vi "Data handler-AOL Zstack.vi"(4 "Save image":bool, 6 "Single Frame Data":T2, 8 "error in (no error)":errorcluster, 9 "Live graph data queue in":T1, 10 "Logging queue element in":T5={"Imaging Protocol"=enum."Live Imaging", "Number of Trials"=0, "Frame Size"=512, "# Averaged frames"=0, "Dwell time (us)"=0.0, "Index of Z-plane"=0, "Timelapse?"=FALSE, "Logging process is active"=FALSE, "Speed logging enabled"=FALSE, "tdms file ref"=refnum, "path"=path "", "Trial Number"=0, "Expected # points acquired"=FALSE, "Manually stopped"=FALSE, "Last trial"=FALSE, "Ch0 data"=[], "Ch1 data"=[], "Image Time"=[], "Continuous Time"=[], "Points acquired"={"Ch0 last trial"=0, "Ch1 last trial"=0, "All trials"=0}, "HW Timings File"=refnum} {"Frame Size" items=["100X100"=100, "128X128"=128, "200X200"=200, "256X256"=256, "512X512"=512, "1024x1024"=1024, "2048x2048"=2048]; "Dwell time (us)" format="%#.6g"}, 11 "Image array":T3) -> (0 "error out":errorcluster)   [LabVIEW 2017]
uses:
  Typedefs/Logging queue element.ctl
  Typedefs/Imaging Protocols enum.ctl
  Typedefs/Frame Size.ctl
  Typedefs/Acquired points count.ctl
  User Interface/Queue/Live graphs queue/Typedefs/Live imaging queue element.ctl
  <vilib>/vision/Image Controls.llb/IMAQ Image.ctl
  Typedefs/Frame data dual cluster.ctl
  User Interface/Typedefs/Live graph data queue ref.ctl
  Typedefs/Subpanel close request.ctl
  Typedefs/Top level VI states.ctl
  Global Variables/General Globals.vi
panel:
  out "Subpanel is closed / Proceed":bool
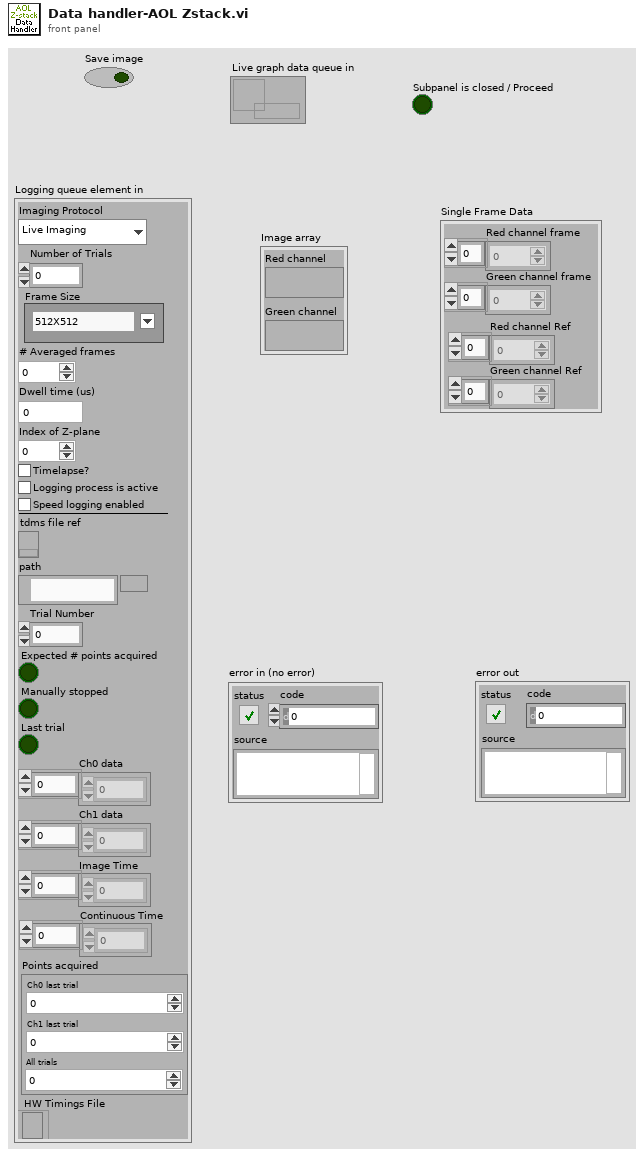
[diagram p1: front panel]
types:
  T1 = typedef "Live graph data queue ref.ctl" = refnum<queue>
  T2 = typedef "Frame data dual cluster.ctl" = cluster{"Red channel frame":dbl[], "Green channel frame":dbl[], "Red channel Ref":dbl[], "Green channel Ref":dbl[]}
  T3 = typedef "Live imaging queue element.ctl" = cluster{"Red channel":T4, "Green channel":T4}
  T4 = typedef "IMAQ Image.ctl" = refnum<image>
  T5 = typedef "Logging queue element.ctl" = cluster{"Imaging Protocol":T6, "Number of Trials":u16, "Frame Size":T7, "# Averaged frames":u16, "Dwell time (us)":dbl, "Index of Z-plane":i32, "Timelapse?":bool, "Logging process is active":bool, "Speed logging enabled":bool, "tdms file ref":refnum<k34>, "path":path, "Trial Number":i32, "Expected # points acquired":bool, "Manually stopped":bool, "Last trial":bool, "Ch0 data":u32[], "Ch1 data":u32[], "Image Time":u64[], "Continuous Time":u64[], "Points acquired":T8, "HW Timings File":refnum<file>}
  T6 = typedef "Imaging Protocols enum.ctl" = enum16{"AOL Z-Stack", "Motor Z Stack", "Functional Acquisition", "Single Plane Acquisition", "Volume Acquisition", "Live Imaging", "Live Plane Imaging", "Live Volume Imaging"}
  T7 = typedef "Frame Size.ctl" = u16
  T8 = typedef "Acquired points count.ctl" = cluster{"Ch0 last trial":u64, "Ch1 last trial":u64, "All trials":u64}
  T9 = typedef "Subpanel close request.ctl" = enum16{"Request subpanel close", "Just check subpanel is closed"}
  T10 = typedef "Top level VI states.ctl" = enum16{"None", "Initialise UI", "<STACK PROTOCOL STATES>", "AOL Zstack-START", "AOL Zstack-STOP", "Motor Zstack-START", "Motor Zstack-STOP", "<ACQUISITION PROTOCOL STATES> ", "Functional Acquisition-START", "Functional Acquisition-STOP", "Single Plane Acquisition-START", "Single Plane Acquisition-STOP", "Volume Acquisition-START", "Volume Acquisition-STOP", "<LIVE IMAGING PROTOCOL STATES>", "Live Imaging-START", "Live Imaging-STOP", "Live Plane Imaging-START", "Live Plane Imaging-STOP", "Live Volume Imaging-START", "Live Volume Imaging-STOP", "<MOVEMENT CORRECTION PROTOCOL STATES>", "EXIT"}
  T11 = enum16{"open", "replace", "create", "open or create", "replace or create", "replace or create with confirmation"}
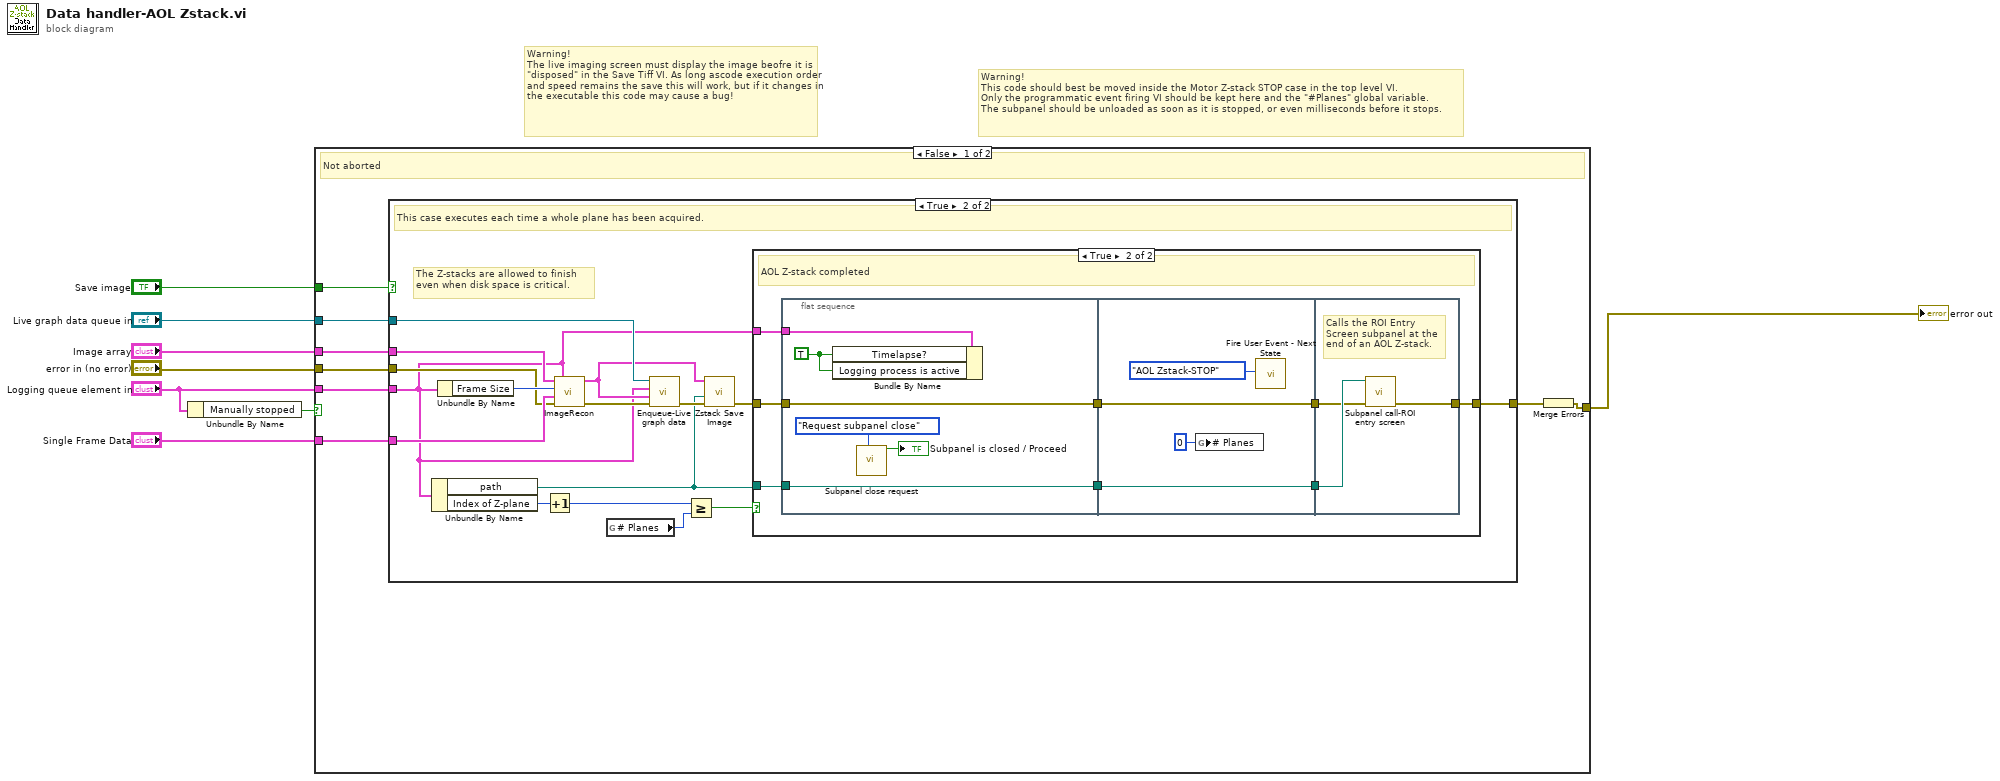
[diagram p0: block diagram]
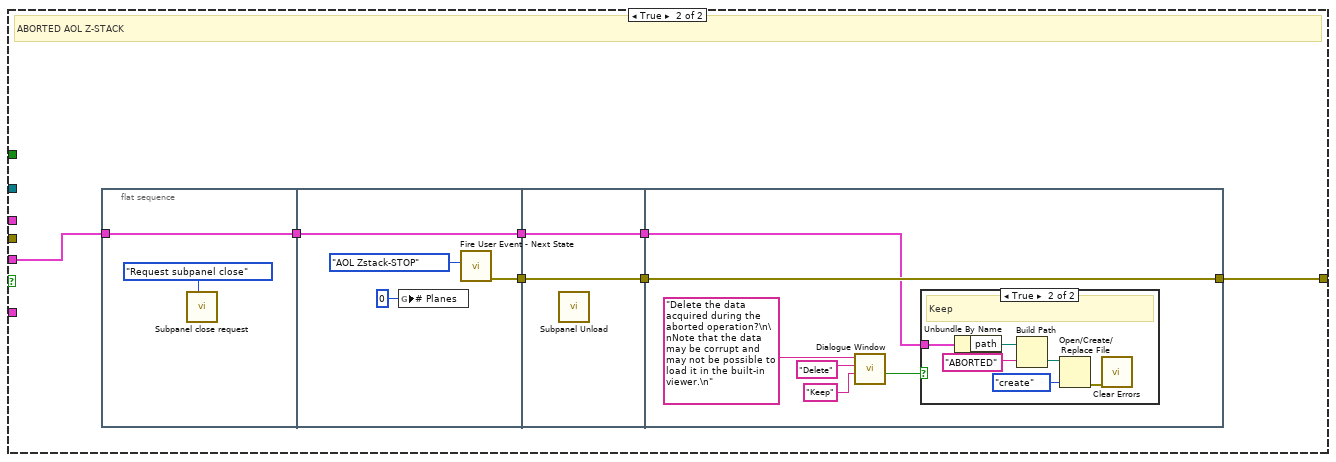
[diagram p4: hidden frame]
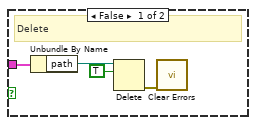
[diagram p5: hidden frame]
diagram:
  # "Warning!\nThe live imaging screen must display the image beofre it is \"disposed\" in the Save Tiff VI. As long ascode execution order and speed remains the save this will work, but if it changes in the executable this code may cause a bug!"
  # "Warning!\nThis code should best be moved inside the Motor Z-stack STOP case in the top level VI.\nOnly the programmatic event firing VI should be kept here and the \"#Planes\" global variable.\nThe subpanel should be unloaded as soon as it is stopped, or even milliseconds before it stops."
  n1 = Unbundle By Name("Logging queue element in") -> ("Manually stopped"=w1:bool)
  n2 = case shown="False" w1 {
    tunnel: "Save image" -> [w15 _]
    tunnel: "error in (no error)" -> [w14 _]
    tunnel: "Live graph data queue in" -> [w13 _]
    tunnel: "Image array" -> [w12 _]
    tunnel: "Single Frame Data" -> [w11 _]
    tunnel: [w10 w61] -> w3
    tunnel: "Logging queue element in" -> [w9 w58]
    frame False {
      # "Not aborted"
      n3 = case shown="True" w15 {
        tunnel: [_ w32] -> w16
        tunnel: w12 -> [_ w30]
        tunnel: w9 -> [_ w18]
        tunnel: w11 -> [_ w27]
        tunnel: w14 -> [_ w26]
        tunnel: w13 -> [_ w25]
        frame False {
          # "Acquisition of the current plane has not completed. Plane is incomplete."
        }
        frame True {
          # "The Z-stacks are allowed to finish even when disk space is critical."
          # "This case executes each time a whole plane has been acquired."
          n4 = Unbundle By Name(w18) -> ("path"=w22:path, "Index of Z-plane"=w28:i32)
          n5 = Unbundle By Name(w18) -> ("Frame Size"=w29:T7)
          n6 = Increment(x=w28) -> (x+1=w31:i32)
          n7 = call "ImageRecon.vi"("Logging queue element in"=w18, "Error In"=w26, "Data"=w27, "Frame Size"=w29, "Image Array (in)"=w30) -> ("Error Out"=w21:errorcluster, "Image Array(out)"=w20:T3)  [unwired: 3 in, 2 out]
          n8 = global read "General Globals.vi" "# Planes"() -> (w19:i32)
          n9 = call "Enqueue-Live graph data.vi"("error in (no error)"=w21, "Element to queue"=w20, "Logging queue element"=w18, "Live graph data queue in"=w25) -> ("error out"=w24:errorcluster)  [unwired: 6 in, 1 out]
          n10 = Greater Or Equal?(x=w31, y=w19) -> (x >= y?=w17:bool)
          n11 = call "Zstack Save Image.vi"("error in (no error)"=w24, "Dataset base-path"=w22, "Image Array"=w20) -> ("error out"=w23:errorcluster)  [unwired: 8 in]
          n12 = case shown="True" w17 {
            tunnel: w23 -> [w33 w39]
            tunnel: w22 -> [_ w41]
            tunnel: [w33 w40] -> w32
            tunnel: w18 -> [_ w34]
            frame False {
            }
            frame True {
              # "AOL Z-stack completed"
              n13 = flat-sequence {
                tunnel: w39 -> [w46]
                tunnel: w41 -> [w47]
                tunnel: [w47] -> w36
                tunnel: [w46] -> w35
                tunnel: w34 -> [w45]
                tunnel: [w51] -> w38
                tunnel: [w48] -> w37
                tunnel: w36 -> [w51]
                tunnel: w35 -> [w48]
                tunnel: [w53] -> w40
                tunnel: w38 -> [w54]
                tunnel: w37 -> [w52]
                frame #0 {
                  w44 = TRUE ("Timelapse?")
                  n14 = Bundle By Name(cluster=w45, "Timelapse?"=w44, "Logging process is active"=w44) -> ()  [unwired: 1 out]
                  n15 = call "Subpanel close request.vi"("Function"=Subpanel_close_request."Request subpanel close") -> ("Subpanel is closed / Proceed"=→"Subpanel is closed / Proceed":bool)  [unwired: 10 in]
                }
                frame #1 {
                  n16 = global write "General Globals.vi" "# Planes"(0 ("# Planes")) -> ()
                  n17 = call "Fire User Event - Next State.vi"("\"UI Handler loop\" case to execute"=Top_level_VI_states."AOL Zstack-STOP" ("event data / imaging mode")) -> ()  [unwired: 10 in, 1 out]
                }
                frame #2 {
                  # "Calls the ROI Entry Screen subpanel at the end of an AOL Z-stack."
                  n18 = call "Subpanel call-ROI entry screen.vi"("error in"=w52, "Experiment folder path"=w54) -> ("error out"=w53:errorcluster)  [unwired: 9 in]
                }
              }
            }
          }
        }
      }
      n19 = Merge Errors(w16) -> (w10:errorcluster)
    }
    frame True {
      # "ABORTED AOL Z-STACK"
      n20 = flat-sequence {
        tunnel: w58 -> [w62]
        tunnel: [w62] -> w57
        tunnel: [w65] -> w60
        tunnel: w57 -> [w64]
        tunnel: [w64] -> w56
        tunnel: w60 -> [w69]
        tunnel: [w69] -> w59
        tunnel: w56 -> [w68]
        tunnel: [w68] -> w55
        tunnel: [w75] -> w61
        tunnel: w59 -> [w75]
        tunnel: w55 -> [w71]
        frame #0 {
          n21 = call "Subpanel close request.vi"("Function"=Subpanel_close_request."Request subpanel close") -> ()  [unwired: 10 in, 1 out]
        }
        frame #1 {
          n22 = global write "General Globals.vi" "# Planes"(0 ("# Planes")) -> ()
          n23 = call "Fire User Event - Next State.vi"("\"UI Handler loop\" case to execute"=Top_level_VI_states."AOL Zstack-STOP" ("event data / imaging mode")) -> ("Error Out"=w65:errorcluster)  [unwired: 10 in]
        }
        frame #2 {
          n24 = call "Subpanel Unload.vi"() -> ()  [unwired: 11 in, 1 out]
        }
        frame #3 {
          n25 = call "Dialogue Window.vi"("Caption-Left button (Cancel)"="Keep", "Caption-Right button (OK)"="Delete", "Message string"="Delete the data acquired during the aborted operation?\n\nNote that the data may be corrupt and may not be possible to load it in the built-in viewer.\n") -> ("Cancelled (Left button pressed)"=w72:bool)  [unwired: 6 in, 2 out]
          n26 = case shown="True" w72 {
            tunnel: w71 -> [w79 w80]
            frame False {
              # "Delete"
              n27 = Unbundle By Name(w79) -> ("path"=w78:path)
              n28 = Delete(path (use dialog)=w78, entire hierarchy (F)=TRUE) -> (error out=w76:errorcluster)  [unwired: 3 in, 2 out]
              n29 = call <vilib>:"Clear Errors.vi"("error in (no error)"=w76) -> ()  [unwired: 5 in, 2 out]
            }
            frame True {
              # "Keep"
              n30 = Unbundle By Name(w80) -> ("path"=w85:path)
              n31 = Build Path(base path=w85, name or relative path="ABORTED") -> (appended path=w82:path)
              n32 = Open/Create/Replace File(file path (use dialog)=w82, operation (0:open)=T11."create") -> (error out=w84:errorcluster)  [unwired: 4 in, 2 out]
              n33 = call <vilib>:"Clear Errors.vi"("error in (no error)"=w84) -> ()  [unwired: 5 in, 2 out]
            }
          }
        }
      }
    }
  }
  "error out" <- w3
